vi "HEWH Agilent Channel List.vi"(8 "error in (no error)":errorcluster) -> (0 "error out":errorcluster, 2 "Analog Channel-List":string)   [LabVIEW 2023]
uses:
  <vilib>/Utility/error.llb/whitespace.ctl
  <vilib>/Utility/error.llb/Trim Whitespace One-Sided.vi
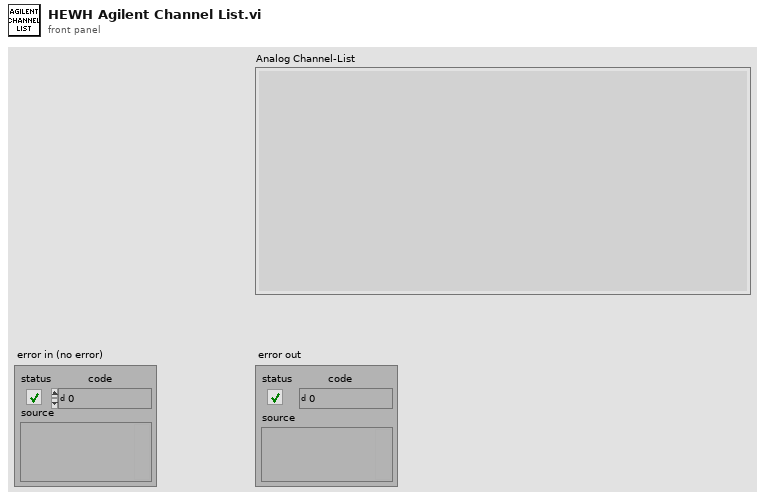
[diagram p1: front panel]
types:
  T1 = typedef "whitespace.ctl" = u16
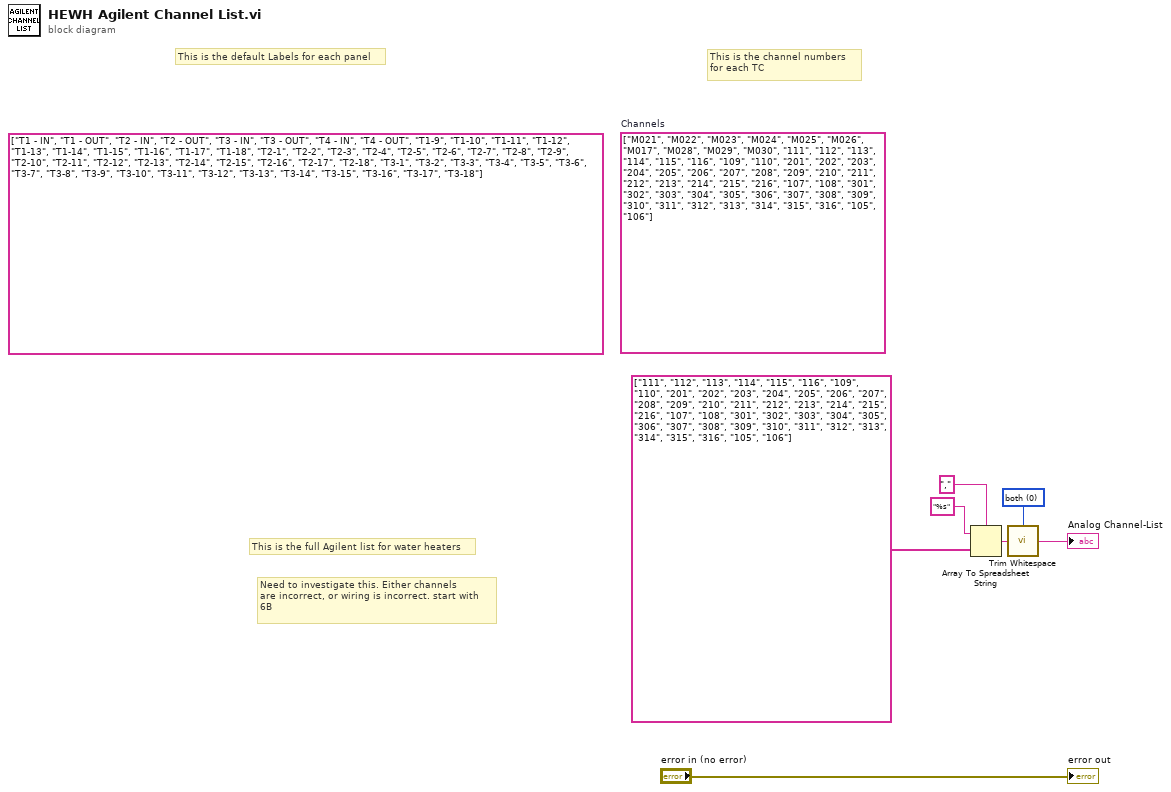
[diagram p0: block diagram]
diagram:
  (unwired) string[][] [["M021", "M022", "M023", "M024", "M025", "M026"], ["M017", "M028", "M029", "M030", "111", "112"], ["113", "114", "115", "116", "109", "110"], ["201", "202", "203", "204", "205", "206"], ["207", "208", "209", "210", "211", "212"], ["213", "214", "215", "216", "107", "108"], ["301", "302", "303", "304", "305", "306"], ["307", "308", "309", "310", "311", "312"], ["313", "314", "315", "316", "105", "106"]]  # Channels
  w3 = T1 0 items=["both", "start of string", "end of string"] ("location (both)")
  (unwired) string[][] [["T1 - IN", "T1 - OUT", "T2 - IN", "T2 - OUT", "T3 - IN", "T3 - OUT"], ["T4 - IN", "T4 - OUT", "T1-9", "T1-10", "T1-11", "T1-12"], ["T1-13", "T1-14", "T1-15", "T1-16", "T1-17", "T1-18"], ["T2-1", "T2-2", "T2-3", "T2-4", "T2-5", "T2-6"], ["T2-7", "T2-8", "T2-9", "T2-10", "T2-11", "T2-12"], ["T2-13", "T2-14", "T2-15", "T2-16", "T2-17", "T2-18"], ["T3-1", "T3-2", "T3-3", "T3-4", "T3-5", "T3-6"], ["T3-7", "T3-8", "T3-9", "T3-10", "T3-11", "T3-12"], ["T3-13", "T3-14", "T3-15", "T3-16", "T3-17", "T3-18"]] ("Array")
  # "Need to investigate this. Either channels\nare incorrect, or wiring is incorrect. start with\n6B"
  # "This is the full Agilent list for water heaters"
  # "This is the channel numbers \nfor each TC"
  # "This is the default Labels for each panel"
  n1 = Array To Spreadsheet String(delimiter (Tab)="," ("format string"), array=string[] ["111", "112", "113", "114", "115", "116", "109", "110", "201", "202", "203", "204", "205", "206", "207", "208", "209", "210", "211", "212", "213", "214", "215", "216", "107", "108", "301", "302", "303", "304", "305", "306", "307", "308", "309", "310", "311", "312", "313", "314", "315", "316", "105", "106"], 3:"%s" ("format string")) -> (spreadsheet string=w4:string)
  n2 = call <vilib>:"Trim Whitespace.vi"("string"=w4, "location (both)"=w3) -> ("trimmed string"=→"Analog Channel-List":string)
  "error out" <- "error in (no error)"
